vi "ReversedEngineering CreateEdges.vi"(1 "NodeRef":refnum<class "AbstractNode.lvclass">, 2 "AllNodes":refnum<class "AbstractNode.lvclass">[](array[class]), 3 "NodeClassInfo":T1, 5 "error in (no error)":errorcluster, 6 "Show Multiplicity":bool=TRUE) -> (15 "EdgesCreated":refnum<class "AbstractEdge.lvclass">[](array[class]), 19 "error out":errorcluster)   [LabVIEW 2020]
uses:
  <resource>/Framework/Providers/Open_GDS/UML/AbstractEdge_class/AbstractEdge.lvclass
  <resource>/Framework/Providers/Open_GDS/UML/AbstractNode_class/AbstractNode.lvclass
  <resource>/Framework/Providers/Open_GDS/UML/ReversedEngineering/ReversedEngineering ClassInfoType.ctl
  <resource>/Framework/Providers/Open_GDS/UML/UMLEditor/UMLEditor_VisibilityType.ctl
  <resource>/Framework/Providers/Open_GDS/UML/ReversedEngineering/ReversedEngineering AttributeInfoType.ctl
  <resource>/Framework/Providers/Open_GDS/ClassProviders/Common/CommonVIs/CommonVIs_AttributeDataType.ctl
  <resource>/Framework/Providers/Open_GDS/UML/ReversedEngineering/ReversedEngineering_ClassDependencyDetailsType.ctl
  <resource>/Framework/Providers/Open_GDS/ClassProviders/Common/ScriptingFunctions/SubVIs/Scripting_ViDependencyType.ctl
  <resource>/Framework/Providers/Open_GDS/UML/ClassRelationshipEdge_class/ClassRelationshipEdge.lvclass
  C:/Program Files (x86)/National Instruments/LabVIEW 2020/resource/Framework/Providers/Open_GDS/UML/AbstractEdge_class/AbstractEdge.lvclass
  <resource>/Framework/Providers/Open_GDS/UML/ClassRelationshipEdge_class/ExternaSetParamType.ctl
  <resource>/Framework/Providers/Open_GDS/UML/ArrowHead_class/ArrowHeadType.ctl
  <resource>/Framework/Providers/Open_GDS/UML/BentStyle_class/BentStyleType.ctl
  <resource>/Framework/Providers/Open_GDS/UML/ReversedEngineering/ReversedEngineering_ViDependencyDetailsType.ctl
  <resource>/Framework/Providers/Open_GDS/UML/ArrowHead_class/ArrowHead.lvclass
  <resource>/Framework/Providers/Open_GDS/UML/BentStyle_class/BentStyle.lvclass
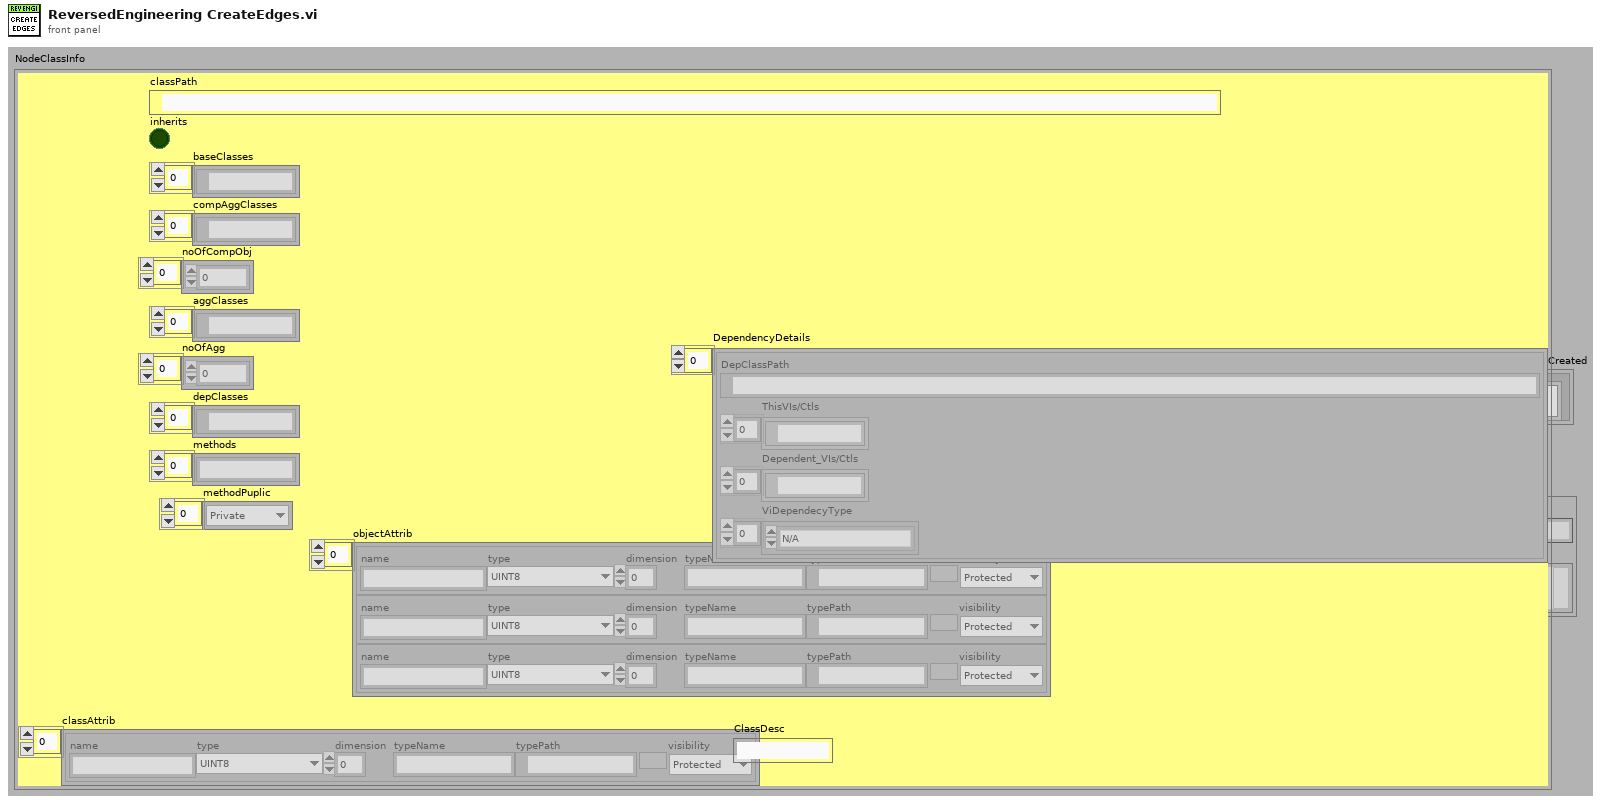
[diagram p1: front panel]
types:
  T1 = typedef "ReversedEngineering ClassInfoType.ctl" = cluster{"classPath":path, "inherits":bool, "baseClasses":path[], "compAggClasses":path[], "noOfCompObj":i32[], "aggClasses":path[], "noOfAgg":i32[], "depClasses":path[], "methods":string[], "methodPuplic":T2[], "objectAttrib":T3[], "classAttrib":T3[], "ClassDesc":string, "DependencyDetails":T5[]}
  T2 = typedef "UMLEditor_VisibilityType.ctl" = enum16{"Public", "Private", "Protected"}
  T3 = typedef "ReversedEngineering AttributeInfoType.ctl" = cluster{"name":string, "type":T4, "dimension":i32, "typeName":string, "typePath":path, "visibility":T2}
  T4 = typedef "CommonVIs_AttributeDataType.ctl" = enum16{"UINT8", "INT8", "UINT16", "INT16", "UINT32", "INT32", "UINT64", "INT64", "SGL", "DBL", "EXT", "CSG", "CDB", "CXT", "TimeStamp", "STRING", "PATH", "BOOL", "ENUM", "RefNum", "VIRefNum", "LabVIEW Class", "Cluster", "Variant", "TypeDef", "Waveform", "LabVIEW Object", "Other", "void"}
  T5 = typedef "ReversedEngineering_ClassDependencyDetailsType.ctl" = cluster{"DepClassPath":path, "ThisVIs/Ctls":path[], "Dependent_VIs/Ctls":path[], "ViDependecyType":T6[]}
  T6 = typedef "Scripting_ViDependencyType.ctl" = enum16{"N/A", "Launches"}
  T7 = typedef "ReversedEngineering_ViDependencyDetailsType.ctl" = cluster{"ThisVIs/Ctls":path[], "Dependent_VIs/Ctls":path[]}
  T8 = typedef "BentStyle.lvclass/BentStyleType.ctl" = enum16{"STRAIGHT", "HV", "VH", "HVH", "VHV", "ARC"}
  T9 = typedef "ClassRelationshipEdge.lvclass/ExternaSetParamType.ctl" = enum16{"StartLabel", "MidLabel", "EndLabel", "StartNode", "EndNode", "BendType", "StartArrow", "EndArrow"}
  T10 = typedef "ArrowHead.lvclass/ArrowHeadType.ctl" = enum16{"NONE", "TRIANGLE", "BLACK_TRIANGLE", "V", "HALF_V", "DIAMOND", "BLACK_DIAMOND"}
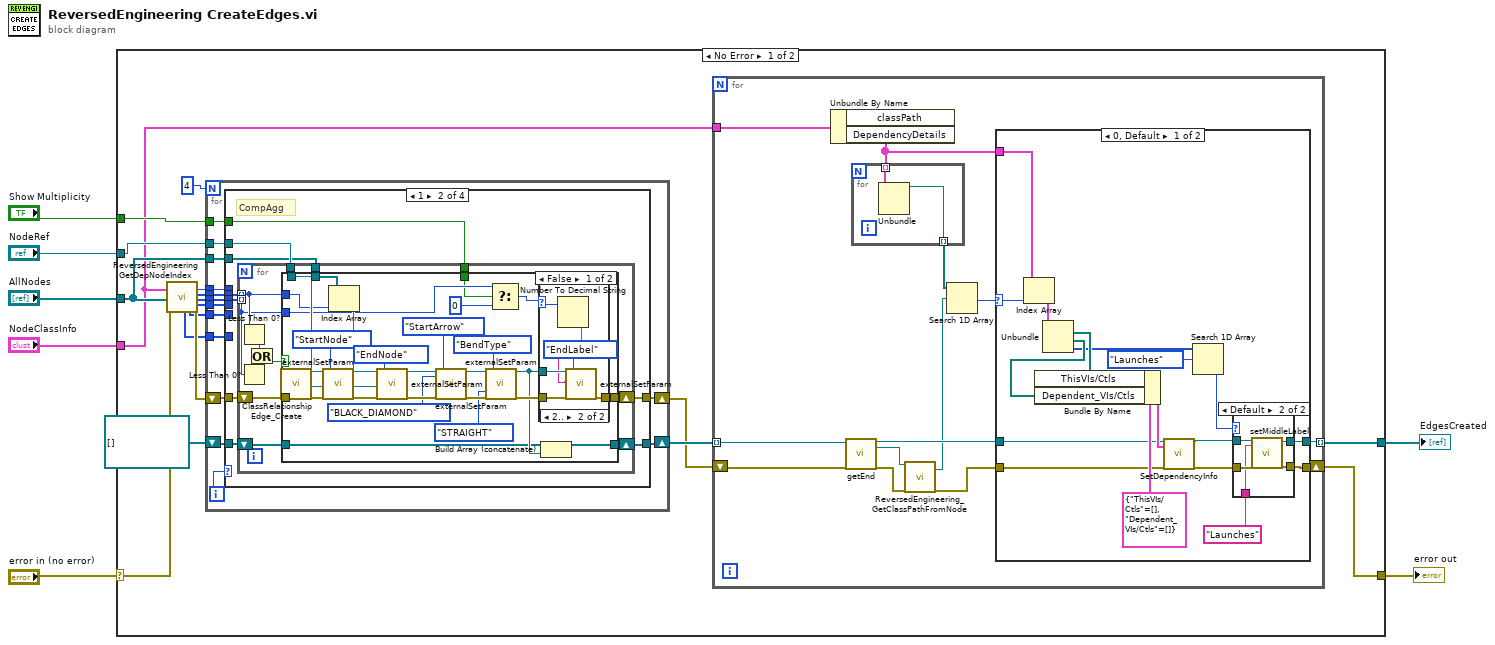
[diagram p0: block diagram]
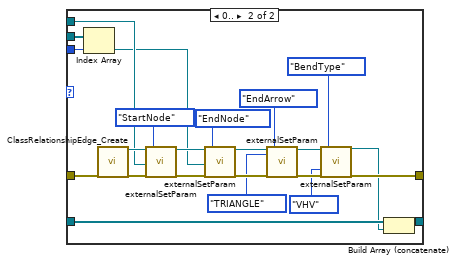
[diagram p5: hidden frame]
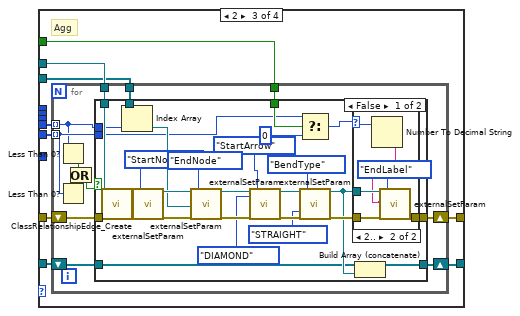
[diagram p8: hidden frame]
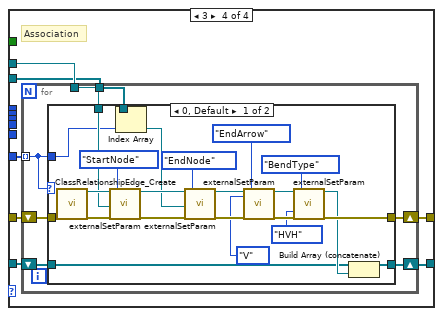
[diagram p11: hidden frame]
diagram:
  n1 = case shown="No Error" "error in (no error)" {
    selector: "error in (no error)" -> [w16 w268]
    tunnel: [w8 w268] -> w6
    tunnel: [w11 _] -> w5
    tunnel: "Show Multiplicity" -> [w15 _]
    tunnel: "AllNodes" -> [w13 _]
    tunnel: "NodeRef" -> [w14 _]
    tunnel: "NodeClassInfo" -> [w10 _]
    frame No Error {
      n2 = call <resource>:"ReversedEngineering GetDepNodeIndex.vi"("classInfo"=w10, "AllNodes"=w13, "error in (no error)"=w16) -> ("depNodes"=w18:i32[], "noOfAgg"=w19:i32[], "inheritanceNode"=w23:i32, "compAggNodes"=w22:i32[], "noOfCompAgg"=w21:i32[], "aggNodes"=w20:i32[], "error out"=w24:errorcluster)  [unwired: 1 in, 9 out]
      n3 = for {
        N: 4 -> [_]
        tunnel: w14 -> [w80]
        shift-right: [w78] -> w9
        shift-left: w24 -> [w79]
        tunnel: w13 -> [w76]
        tunnel: w23 -> [w75]
        shift-right: [w74] -> w12
        shift-left: refnum<class "ClassRelationshipEdge.lvclass">[] [] ("empty") -> [w73]
        tunnel: w22 -> [w72]
        tunnel: w21 -> [w71]
        tunnel: w20 -> [w70]
        tunnel: w19 -> [w69]
        tunnel: w18 -> [w68]
        tunnel: w15 -> [w67]
        i -> [w77]
        n4 = case shown="1" w77 {
          tunnel: w79 -> [w87 w121 w179 w235]
          tunnel: w80 -> [w86 w120 w178 w234]
          tunnel: [w82 w119 w177 w233] -> w78
          tunnel: w76 -> [w85 w117 w176 w232]
          tunnel: w75 -> [w81 _ _ _]
          tunnel: [w84 w114 w174 w230] -> w74
          tunnel: w73 -> [w83 w115 w175 w231]
          tunnel: w72 -> [_ w118 _ _]
          tunnel: w71 -> [_ w116 _ _]
          tunnel: w70 -> [_ _ w173 _]
          tunnel: w69 -> [_ _ w172 _]
          tunnel: w68 -> [_ _ _ w229]
          tunnel: w67 -> [_ w113 w171 _]
          frame 0, Default {
            # "Inheritance"
            n5 = case shown="Default" w81 {
              tunnel: w87 -> [w89 w112]
              tunnel: w86 -> [_ w103]
              tunnel: w85 -> [_ w102]
              tunnel: w81 -> [_ w101]
              tunnel: [w88 w97] -> w84
              tunnel: w83 -> [w88 w96]
              tunnel: [w89 w93] -> w82
              frame Default {
              }
              frame 0.. {
                n6 = Index Array(array=w102, index=w101) -> (element=w100:refnum<class "AbstractNode.lvclass">)
                n7 = call <resource>:"ClassRelationshipEdge_Create.vi"("error in (no error)"=w112) -> ("reference out"=w111:refnum<class "ClassRelationshipEdge.lvclass">, "error out"=w110:errorcluster)  [unwired: 1 in, 16 out]
                n8 = call-dynamic "externalSetParam.vi"("reference"=w111, "node"=w103, "error in (no error)"=w110, "setParam"=ExternaSetParamType."StartNode") -> ("reference out"=w108:refnum<class "ClassRelationshipEdge.lvclass">, "error out"=w107:errorcluster)  [unwired: 14 in]
                n9 = call-dynamic "externalSetParam.vi"("reference"=w108, "node"=w100, "error in (no error)"=w107, "setParam"=ExternaSetParamType."EndNode") -> ("reference out"=w106:refnum<class "ClassRelationshipEdge.lvclass">, "error out"=w105:errorcluster)  [unwired: 14 in]
                n10 = call-dynamic "externalSetParam.vi"("reference"=w106, "arrowHead"=ArrowHeadType."TRIANGLE", "error in (no error)"=w105, "setParam"=ExternaSetParamType."EndArrow") -> ("reference out"=w95:refnum<class "ClassRelationshipEdge.lvclass">, "error out"=w94:errorcluster)  [unwired: 14 in]
                n11 = call-dynamic "externalSetParam.vi"("reference"=w95, "bentStyle"=BentStyleType."VHV", "error in (no error)"=w94, "setParam"=ExternaSetParamType."BendType") -> ("reference out"=w92:refnum<class "ClassRelationshipEdge.lvclass">, "error out"=w93:errorcluster)  [unwired: 14 in]
                n12 = Build Array (concatenate)(w96, w92) -> (w97:refnum<class "ClassRelationshipEdge.lvclass">[])
              }
            }
          }
          frame 1 {
            # "CompAgg"
            n13 = for {
              shift-right: [w131] -> w119
              shift-left: w121 -> [w133]
              tunnel: w120 -> [w132]
              tunnel: w118 -> [w126] mode=indexing
              tunnel: w117 -> [w130]
              tunnel: w116 -> [w125] mode=indexing
              shift-right: [w128] -> w114
              shift-left: w115 -> [w129]
              tunnel: w113 -> [w127]
              n14 = Less Than 0?(x=w126) -> (x < 0?=w124:bool)
              n15 = Less Than 0?(x=w125) -> (x < 0?=w123:bool)
              n16 = Or(x=w124, y=w123) -> (x .or. y?=w122:bool)
              n17 = case shown="False" w122 {
                tunnel: w133 -> [w150 w170]
                tunnel: w132 -> [w149 _]
                tunnel: [w148 w170] -> w131
                tunnel: w126 -> [w147 _]
                tunnel: w130 -> [w146 _]
                tunnel: w129 -> [w140 w169]
                tunnel: [w139 w169] -> w128
                tunnel: w125 -> [w136 _]
                tunnel: w127 -> [w135 _]
                frame False {
                  n18 = call <resource>:"ClassRelationshipEdge_Create.vi"("error in (no error)"=w150) -> ("reference out"=w161:refnum<class "ClassRelationshipEdge.lvclass">, "error out"=w160:errorcluster)  [unwired: 1 in, 16 out]
                  n19 = call-dynamic "externalSetParam.vi"("reference"=w161, "node"=w149, "error in (no error)"=w160, "setParam"=ExternaSetParamType."StartNode") -> ("reference out"=w158:refnum<class "ClassRelationshipEdge.lvclass">, "error out"=w157:errorcluster)  [unwired: 14 in]
                  n20 = Index Array(array=w146, index=w147) -> (element=w145:refnum<class "AbstractNode.lvclass">)
                  n21 = call-dynamic "externalSetParam.vi"("reference"=w158, "node"=w145, "error in (no error)"=w157, "setParam"=ExternaSetParamType."EndNode") -> ("reference out"=w156:refnum<class "ClassRelationshipEdge.lvclass">, "error out"=w155:errorcluster)  [unwired: 14 in]
                  n22 = call-dynamic "externalSetParam.vi"("reference"=w156, "arrowHead"=ArrowHeadType."BLACK_DIAMOND", "error in (no error)"=w155, "setParam"=ExternaSetParamType."StartArrow") -> ("reference out"=w154:refnum<class "ClassRelationshipEdge.lvclass">, "error out"=w153:errorcluster)  [unwired: 14 in]
                  n23 = call-dynamic "externalSetParam.vi"("reference"=w154, "bentStyle"=BentStyleType."STRAIGHT", "error in (no error)"=w153, "setParam"=ExternaSetParamType."BendType") -> ("reference out"=w141:refnum<class "ClassRelationshipEdge.lvclass">, "error out"=w152:errorcluster)  [unwired: 14 in]
                  n24 = Select(t=w136, s=w135, f=0) -> (s? t:f=w137:i32)
                  n25 = case shown="2.." w137 {
                    selector: w137 -> [_ w165]
                    tunnel: w141 -> [_ w168]
                    tunnel: w152 -> [w162 w167]
                    tunnel: [w162 w166] -> w148
                    frame 0, Default {
                    }
                    frame 2.. {
                      n26 = Number To Decimal String(number=w165) -> (decimal integer string=w164:string)  [unwired: 1 out]
                      n27 = call-dynamic "externalSetParam.vi"("reference"=w168, "string"=w164, "error in (no error)"=w167, "setParam"=ExternaSetParamType."EndLabel") -> ("error out"=w166:errorcluster)  [unwired: 14 in, 1 out]
                    }
                  }
                  n28 = Build Array (concatenate)(w140, w141) -> (w139:refnum<class "ClassRelationshipEdge.lvclass">[])
                }
                frame True {
                }
              }
            }
          }
          frame 2 {
            # "Agg"
            n29 = for {
              shift-right: [w189] -> w177
              shift-left: w179 -> [w191]
              tunnel: w178 -> [w190]
              tunnel: w173 -> [w181] mode=indexing
              tunnel: w176 -> [w188]
              tunnel: w172 -> [w182] mode=indexing
              shift-right: [w186] -> w174
              shift-left: w175 -> [w187]
              tunnel: w171 -> [w185]
              n30 = Less Than 0?(x=w181) -> (x < 0?=w184:bool)
              n31 = Less Than 0?(x=w182) -> (x < 0?=w183:bool)
              n32 = Or(x=w184, y=w183) -> (x .or. y?=w180:bool)
              n33 = case shown="False" w180 {
                tunnel: w191 -> [w208 w228]
                tunnel: w190 -> [w207 _]
                tunnel: [w206 w228] -> w189
                tunnel: w188 -> [w205 _]
                tunnel: w187 -> [w198 w227]
                tunnel: [w197 w227] -> w186
                tunnel: w185 -> [w194 _]
                tunnel: w182 -> [w193 _]
                tunnel: w181 -> [w192 _]
                frame False {
                  n34 = call <resource>:"ClassRelationshipEdge_Create.vi"("error in (no error)"=w208) -> ("reference out"=w219:refnum<class "ClassRelationshipEdge.lvclass">, "error out"=w218:errorcluster)  [unwired: 1 in, 16 out]
                  n35 = Index Array(array=w205, index=w192) -> (element=w204:refnum<class "AbstractNode.lvclass">)
                  n36 = call-dynamic "externalSetParam.vi"("reference"=w219, "node"=w207, "error in (no error)"=w218, "setParam"=ExternaSetParamType."StartNode") -> ("reference out"=w216:refnum<class "ClassRelationshipEdge.lvclass">, "error out"=w215:errorcluster)  [unwired: 14 in]
                  n37 = call-dynamic "externalSetParam.vi"("reference"=w216, "node"=w204, "error in (no error)"=w215, "setParam"=ExternaSetParamType."EndNode") -> ("reference out"=w214:refnum<class "ClassRelationshipEdge.lvclass">, "error out"=w213:errorcluster)  [unwired: 14 in]
                  n38 = call-dynamic "externalSetParam.vi"("reference"=w214, "arrowHead"=ArrowHeadType."DIAMOND", "error in (no error)"=w213, "setParam"=ExternaSetParamType."StartArrow") -> ("reference out"=w212:refnum<class "ClassRelationshipEdge.lvclass">, "error out"=w211:errorcluster)  [unwired: 14 in]
                  n39 = Select(t=w193, s=w194, f=0) -> (s? t:f=w195:i32)
                  n40 = call-dynamic "externalSetParam.vi"("reference"=w212, "bentStyle"=BentStyleType."STRAIGHT", "error in (no error)"=w211, "setParam"=ExternaSetParamType."BendType") -> ("reference out"=w199:refnum<class "ClassRelationshipEdge.lvclass">, "error out"=w210:errorcluster)  [unwired: 14 in]
                  n41 = case shown="2.." w195 {
                    selector: w195 -> [_ w223]
                    tunnel: w199 -> [_ w226]
                    tunnel: w210 -> [w220 w225]
                    tunnel: [w220 w224] -> w206
                    frame 0, Default {
                    }
                    frame 2.. {
                      n42 = Number To Decimal String(number=w223) -> (decimal integer string=w222:string)  [unwired: 1 out]
                      n43 = call-dynamic "externalSetParam.vi"("reference"=w226, "string"=w222, "error in (no error)"=w225, "setParam"=ExternaSetParamType."EndLabel") -> ("error out"=w224:errorcluster)  [unwired: 14 in, 1 out]
                    }
                  }
                  n44 = Build Array (concatenate)(w198, w199) -> (w197:refnum<class "ClassRelationshipEdge.lvclass">[])
                }
                frame True {
                }
              }
            }
          }
          frame 3 {
            # "Association"
            n45 = for {
              shift-right: [w240] -> w233
              shift-left: w235 -> [w242]
              tunnel: w234 -> [w241]
              tunnel: w232 -> [w239]
              shift-right: [w237] -> w230
              shift-left: w231 -> [w238]
              tunnel: w229 -> [w236] mode=indexing
              n46 = case shown="0, Default" w236 {
                tunnel: w242 -> [w255 w267]
                tunnel: w241 -> [w254 _]
                tunnel: [w253 w267] -> w240
                tunnel: w239 -> [w252 _]
                tunnel: w238 -> [w245 w266]
                tunnel: [w244 w266] -> w237
                tunnel: w236 -> [w243 _]
                frame 0, Default {
                  n47 = call <resource>:"ClassRelationshipEdge_Create.vi"("error in (no error)"=w255) -> ("reference out"=w265:refnum<class "ClassRelationshipEdge.lvclass">, "error out"=w264:errorcluster)  [unwired: 1 in, 16 out]
                  n48 = call-dynamic "externalSetParam.vi"("reference"=w265, "node"=w254, "error in (no error)"=w264, "setParam"=ExternaSetParamType."StartNode") -> ("reference out"=w262:refnum<class "ClassRelationshipEdge.lvclass">, "error out"=w261:errorcluster)  [unwired: 14 in]
                  n49 = Index Array(array=w252, index=w243) -> (element=w251:refnum<class "AbstractNode.lvclass">)
                  n50 = call-dynamic "externalSetParam.vi"("reference"=w262, "node"=w251, "error in (no error)"=w261, "setParam"=ExternaSetParamType."EndNode") -> ("reference out"=w260:refnum<class "ClassRelationshipEdge.lvclass">, "error out"=w259:errorcluster)  [unwired: 14 in]
                  n51 = call-dynamic "externalSetParam.vi"("reference"=w260, "arrowHead"=ArrowHeadType."V", "error in (no error)"=w259, "setParam"=ExternaSetParamType."EndArrow") -> ("reference out"=w258:refnum<class "ClassRelationshipEdge.lvclass">, "error out"=w257:errorcluster)  [unwired: 14 in]
                  n52 = call-dynamic "externalSetParam.vi"("reference"=w258, "bentStyle"=BentStyleType."HVH", "error in (no error)"=w257, "setParam"=ExternaSetParamType."BendType") -> ("reference out"=w246:refnum<class "ClassRelationshipEdge.lvclass">, "error out"=w253:errorcluster)  [unwired: 14 in]
                  n53 = Build Array (concatenate)(w245, w246) -> (w244:refnum<class "ClassRelationshipEdge.lvclass">[])
                }
                frame -1 {
                }
              }
            }
          }
        }
      }
      n54 = for {
        tunnel: w12 -> [w26] mode=indexing
        tunnel: [w37] -> w11 mode=indexing
        tunnel: w10 -> [w38]
        shift-right: [w36] -> w8
        shift-left: w9 -> [w27]
        n55 = Unbundle By Name(w38) -> ("DependencyDetails"=w28:T5[])  [unwired: 1 out]
        n56 = call-dynamic "getEnd.vi"("reference"=w26, "error in (no error)"=w27) -> ("reference out"=w33:refnum<class "ClassRelationshipEdge.lvclass">, "endNode"=w34:refnum<class "AbstractNode.lvclass">, "error out"=w35:errorcluster)  [unwired: 14 in, 1 out]
        n57 = for {
          tunnel: w28 -> [w66] mode=indexing
          tunnel: [w65] -> w32 mode=indexing
          n58 = Unbundle(w66) -> ("DepClassPath"=w65:path)  [unwired: 3 out]
        }
        n59 = call <resource>:"ReversedEngineering_GetClassPathFromNode.vi"("reference"=w34, "error IO"=w35) -> ("Path"=w31:path, "error out"=w29:errorcluster)  [unwired: 2 in, 14 out]
        n60 = Search 1D Array(1D array=w32, element=w31) -> (index of element=w30:i32)  [unwired: 1 out]
        n61 = case shown="0, Default" w30 {
          selector: w30 -> [w51 _]
          tunnel: [w41 w64] -> w37
          tunnel: [w42 w63] -> w36
          tunnel: w33 -> [w53 w64]
          tunnel: w29 -> [w52 w63]
          tunnel: w28 -> [w50 _]
          frame 0, Default {
            n62 = Index Array(array=w50, index=w51) -> (element=w49:T5)
            n63 = Unbundle(w49) -> ("ThisVIs/Ctls"=w48:path[], "Dependent_VIs/Ctls"=w47:path[], "ViDependecyType"=w46:T6[])  [unwired: 1 out]
            n64 = Bundle By Name(cluster=T7 {"ThisVIs/Ctls"=[], "Dependent_VIs/Ctls"=[]} ("DepClass"), "ThisVIs/Ctls"=w48, "Dependent_VIs/Ctls"=w47) -> (w54:T7)
            n65 = call <resource>:"SetDependencyInfo.vi"("reference"=w53, "DepClass"=w54, "error in (no error)"=w52) -> ("reference out"=w44:refnum<class "ClassRelationshipEdge.lvclass">, "error out"=w43:errorcluster)  [unwired: 15 out]
            n66 = Search 1D Array(1D array=w46, element=Scripting_ViDependencyType."Launches") -> (index of element=w40:i32)  [unwired: 1 in]
            n67 = case shown="Default" w40 {
              tunnel: w44 -> [w57 w62]
              tunnel: w43 -> [w56 w61]
              tunnel: [w56 w60] -> w42
              tunnel: [w57 w59] -> w41
              tunnel: "Launches" ("middleLabel") -> [_ w58]
              frame -1 {
              }
              frame Default {
                n68 = call-dynamic "setMiddleLabel.vi"("reference"=w62, "middleLabel"=w58, "error in (no error)"=w61) -> ("reference out"=w59:refnum<class "ClassRelationshipEdge.lvclass">, "error out"=w60:errorcluster)  [unwired: 15 in]
              }
            }
          }
          frame -1 {
          }
        }
      }
    }
    frame Error {
    }
  }
  "error out" <- w6
  "EdgesCreated" <- w5
